vi "VIS-IR_SRingStartFetch.vi"(8 "error in (no error)":errorcluster, 11 "VIS-IR in":refnum<class "VIS-NIR.lvclass">) -> (0 "error out":errorcluster, 3 "VIS-IR out":refnum<class "VIS-NIR.lvclass">)   [LabVIEW 2015, in "VIS-NIR.lvclass"]
uses:
  VIS-NIR.lvclass
  Detector.lvclass/Detector.ctl
  Detector.lvclass
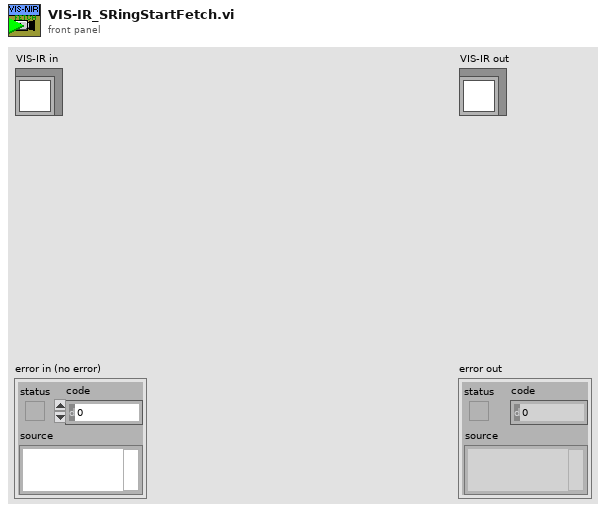
[diagram p1: front panel]
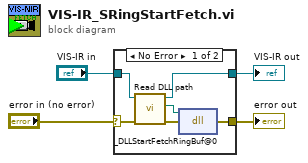
[diagram p0: block diagram]
diagram:
  n1 = case shown="No Error" "error in (no error)" {
    selector: "error in (no error)" -> [w9 w12]
    tunnel: [w7 w12] -> w3
    tunnel: [w5 w11] -> w1
    tunnel: "VIS-IR in" -> [w10 w11]
    frame No Error {
      n2 = call "Read DLL path.vi"("error in (no error)"=w9, "Detector in"=w10) -> ("error out"=w8:errorcluster, "DLL path"=w6:path, "Detector out"=w5:refnum<class "VIS-NIR.lvclass">)  [unwired: 7 in]
      n3 = dll-call lib="G:/SD/TRANCON/DLL/ESLSCDLL.dll" fn="_DLLStartFetchRingBuf@0" ("lwlscdll.dll:DLLStartFetchRingBuf")(path in=w6, error in=w8) -> (error out=w7:errorcluster)  [unwired: 2 in, 1 out]
    }
    frame Error {
    }
  }
  "error out" <- w3
  "VIS-IR out" <- w1
